vi "Tavle Save Conver to PD .vi"(8 "error in (no error)":errorcluster, 11 "SN":string="012345678911111111112") -> (0 "error out 2":errorcluster)   [LabVIEW 2019]
uses:
  Ctrl/Table Save.ctl
  Ctrl/MeasureDisplayTab.ctl
  Ctrl/PD Table Save Low Index.ctl
  Ctrl/PD Table Save Col Index.ctl
  <vilib>/Utility/sysdir.llb/System Directory Type.ctl
  <vilib>/Utility/file.llb/Read Delimited Spreadsheet (string).vi
  <vilib>/Utility/file.llb/Write Delimited Spreadsheet (string).vi
panel:
  out "硬體":string
  out "Read SN Table":string[][](array[string])
  out "first row":string[](array[string])
  out "all rows":string[][](array[string])
  out "error out":errorcluster
  in  "Read SN Table 2":string[][](array[string])
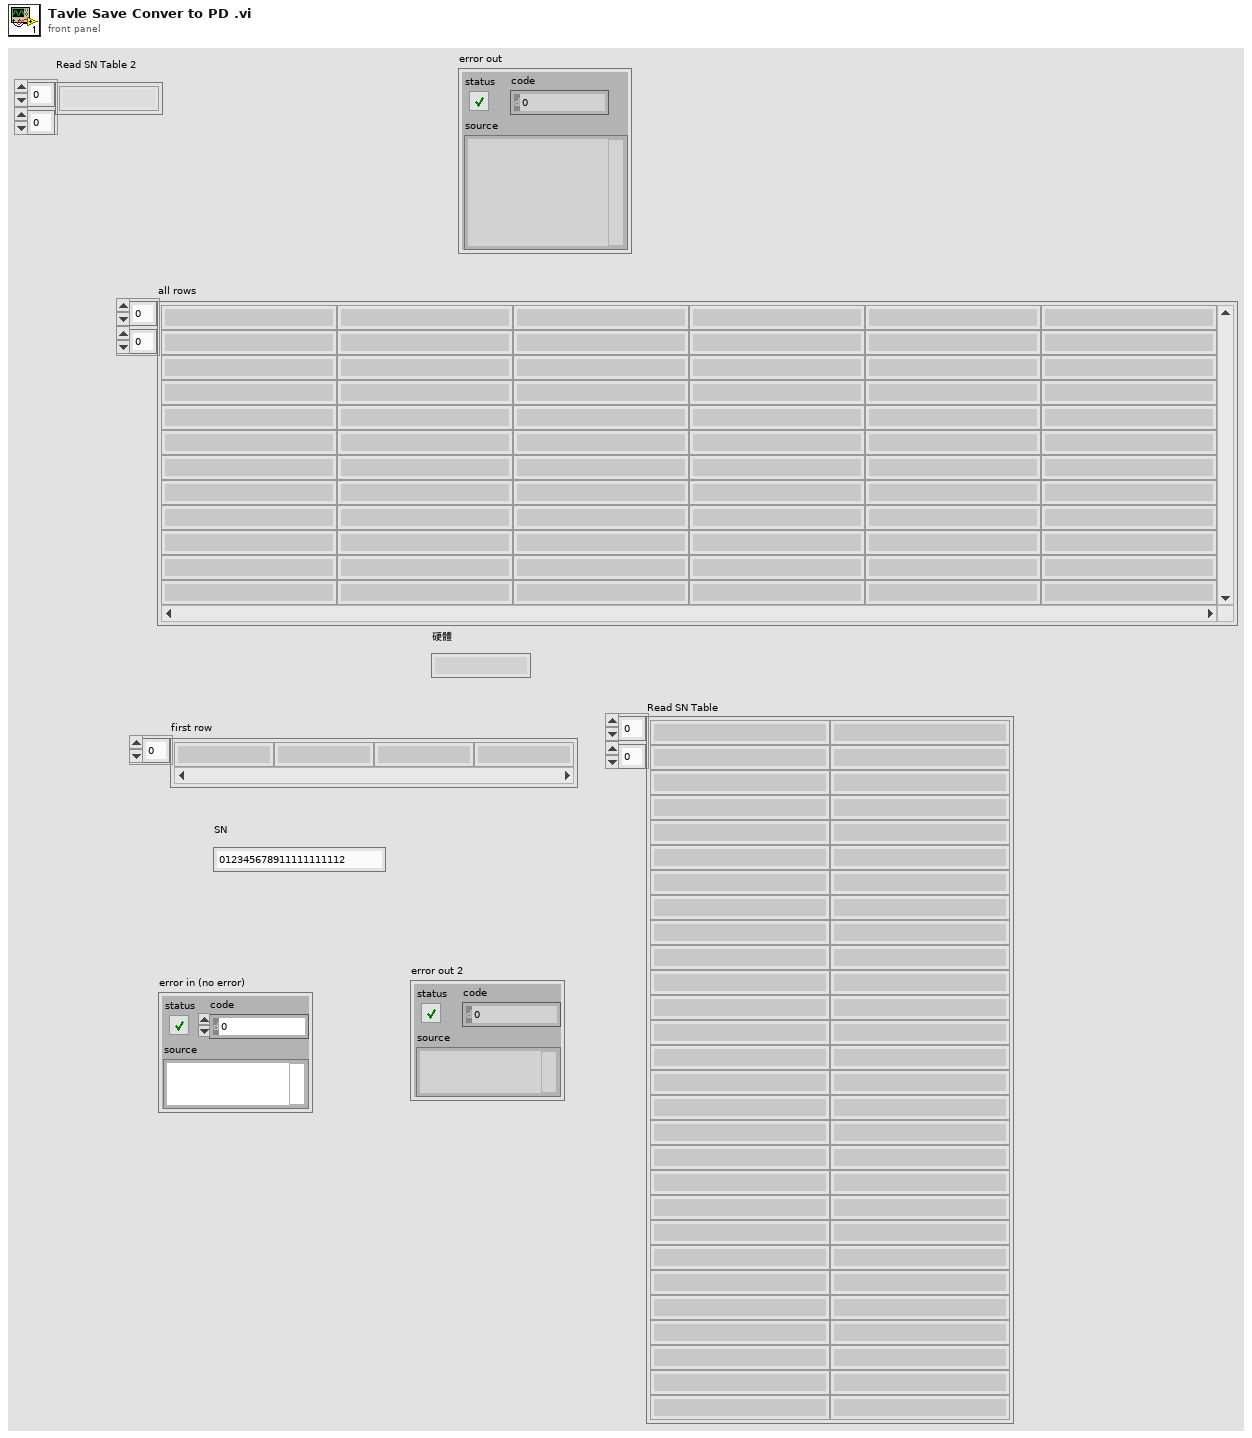
[diagram p1: front panel]
types:
  T1 = typedef "Table Save.ctl" = enum16{"initial", "Add", "Write", "Replace", "Delete", "REad", "RedTable", "Load"}
  T2 = typedef "MeasureDisplayTab.ctl" = enum16{"Tray Barcode", "PCBA BARCODE", "硬體(Tool初始化)", "company(Tool初始化)", "耗電流 uA(電流表)", "電池負載電壓", "晶片ID(Tool FORMAT)", "雷雕ID(TOOl scan、藍芽接收器)", "Format(Tool FORMAT)", "Programe(Tool Programe)", "MAC(藍芽接收器)", "ID(藍芽接收器)", "KPA(藍芽接收器)", "溫度(藍芽接收器)", "SENSOR電池電壓(藍芽接收器)", "RSSI(藍芽接收器)", "SensorType_315(FSK scan)", "FSKsnVol_315(FSK scan)", "FSKscanl_315(FSK scan)", "P_315(FSK scan)", "T_315(FSK scan)", "SensorType_433(ASK scan)", "ASKsnVol_433(ASK scan)", "ASKscan_433(ASK scan)", "P_433(ASK scan)", "T_433(ASK scan)", "測高Data"}
  T3 = typedef "PD Table Save Col Index.ctl" = enum16{"Col A", "Col B", "PCBA SN_C", "scan 半成品 ID_1_D", "半成品 Waste_Time_E", "半成品 Result_F", "半成品 DateTime_G", "433半成品 版本_H", "433半成品 company_I", "433半成品 FF_J", "433半成品 SensorType_K", "433半成品 BattVol_L", "433半成品 ASKsnVOL_M", "433半成品 ID_2_N", "433半成品 Format_O", "433半成品 Programe_P", "433半成品 ASKscan_Q", "433半成品 FSKscan_R", "433半成品 Batt_S", "433半成品 SN_T", "433半成品 Ptest_U", "433半成品 Ttest_V", "433半成品 P_W", "433半成品 T_X", "433半成品 結果_Y", "433半成品 箱號_Z", "不良代碼_AA", "電流_AB", "電池電壓_AC", "315半成品 版本_AD", "315半成品 company_AE", "315半成品 FF_AF", "315半成品 SensorType_AG", "315半成品 BattVol_AH", "315半成品 ASKsnVOL_AI", "315半成品 ID_2_AJ", "315半成品 Format_AK", "315半成品 Programe_AL", "315半成品 ASKscan_AM", "315半成品 FSKscan_AN", "315半成品 Batt_AO", "315半成品 SN_AP", "315半成品 Ptest_AQ", "315半成品 Ttest_AR", "315半成品 P_AS", "315半成品 T_AT"}
  T4 = typedef "PD Table Save Low Index.ctl" = enum16{"low 1", "low 2", "low 3", "low 4", "一般模式F", "一般模式P", "一般模式S", "low 8", "藍芽模式F", "藍芽模式P", "藍芽模式S"}
  T5 = typedef "System Directory Type.ctl" = i32
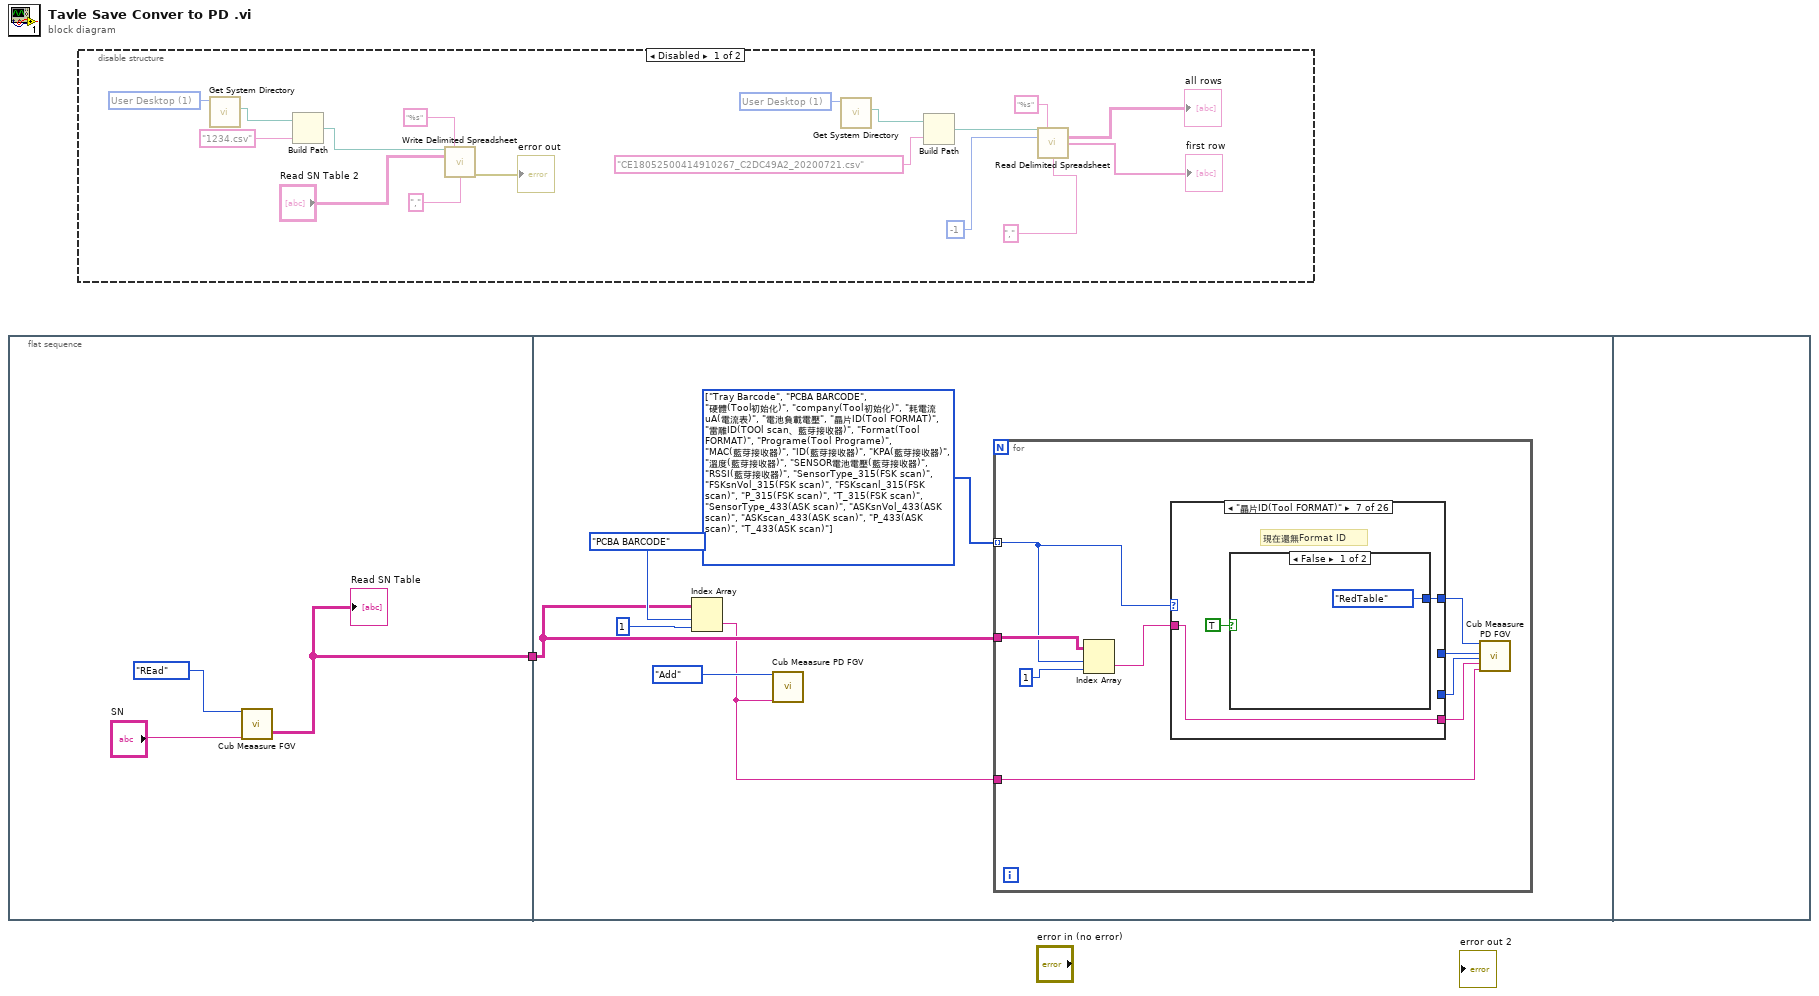
[diagram p0: block diagram]
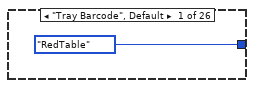
[diagram p3: hidden frame]
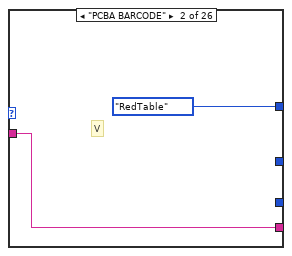
[diagram p4: hidden frame]
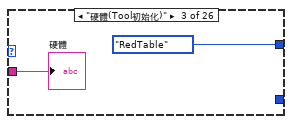
[diagram p5: hidden frame]
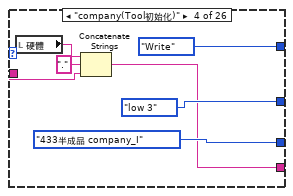
[diagram p6: hidden frame]
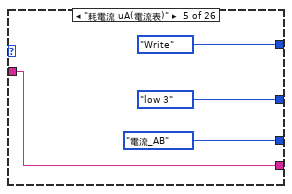
[diagram p7: hidden frame]
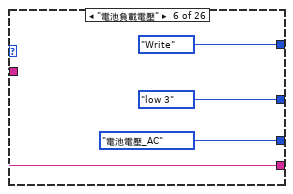
[diagram p8: hidden frame]
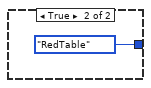
[diagram p9: hidden frame]
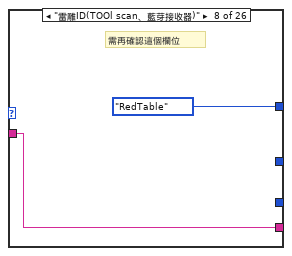
[diagram p10: hidden frame]
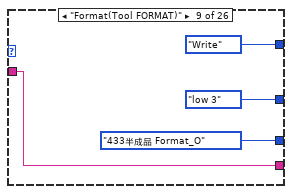
[diagram p11: hidden frame]
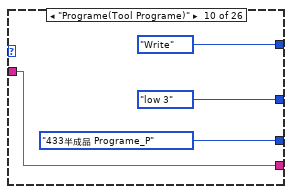
[diagram p12: hidden frame]
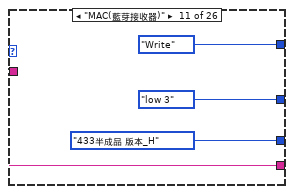
[diagram p13: hidden frame]
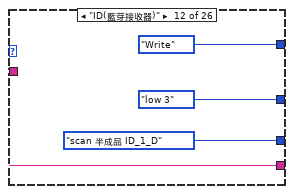
[diagram p14: hidden frame]
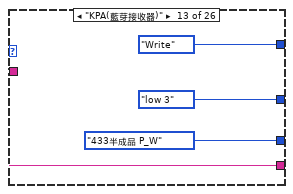
[diagram p15: hidden frame]
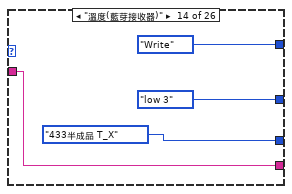
[diagram p16: hidden frame]
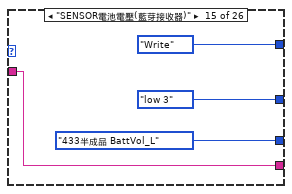
[diagram p17: hidden frame]
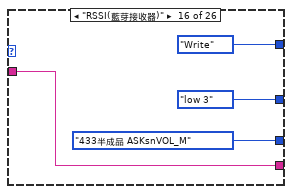
[diagram p18: hidden frame]
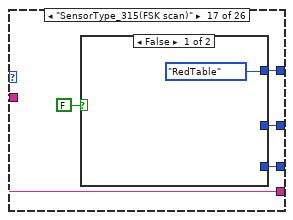
[diagram p19: hidden frame]
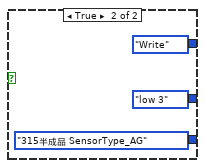
[diagram p20: hidden frame]
diagram:
  n1 = flat-sequence {
    tunnel: [w3] -> w1
    tunnel: w1 -> [w7]
    frame #0 {
      n2 = call "Cub Meaasure FGV.vi"("Action"=Table_Save."REad", "SN"="SN") -> ("Read SN Table"=w3:string[][])  [unwired: 10 in, 7 out]
      "Read SN Table" <- w3
    }
    frame #1 {
      w5 = T2[] [enum."Tray Barcode", enum."PCBA BARCODE", enum."硬體(Tool初始化)", enum."company(Tool初始化)", enum."耗電流 uA(電流表)", enum."電池負載電壓", enum."晶片ID(Tool FORMAT)", enum."雷雕ID(TOOl scan、藍芽接收器)", enum."Format(Tool FORMAT)", enum."Programe(Tool Programe)", enum."MAC(藍芽接收器)", enum."ID(藍芽接收器)", enum."KPA(藍芽接收器)", enum."溫度(藍芽接收器)", enum."SENSOR電池電壓(藍芽接收器)", enum."RSSI(藍芽接收器)", enum."SensorType_315(FSK scan)", enum."FSKsnVol_315(FSK scan)", enum."FSKscanl_315(FSK scan)", enum."P_315(FSK scan)", enum."T_315(FSK scan)", enum."SensorType_433(ASK scan)", enum."ASKsnVol_433(ASK scan)", enum."ASKscan_433(ASK scan)", enum."P_433(ASK scan)", enum."T_433(ASK scan)"] items=["Tray Barcode", "PCBA BARCODE", "硬體(Tool初始化)", "company(Tool初始化)", "耗電流 uA(電流表)", "電池負載電壓", "晶片ID(Tool FORMAT)", "雷雕ID(TOOl scan、藍芽接收器)", "Format(Tool FORMAT)", "Programe(Tool Programe)", "MAC(藍芽接收器)", "ID(藍芽接收器)", "KPA(藍芽接收器)", "溫度(藍芽接收器)", "SENSOR電池電壓(藍芽接收器)", "RSSI(藍芽接收器)", "SensorType_315(FSK scan)", "FSKsnVol_315(FSK scan)", "FSKscanl_315(FSK scan)", "P_315(FSK scan)", "T_315(FSK scan)", "SensorType_433(ASK scan)", "ASKsnVol_433(ASK scan)", "ASKscan_433(ASK scan)", "P_433(ASK scan)", "T_433(ASK scan)", "測高Data"]
      n3 = Index Array(array=w7, index (row)=MeasureDisplayTab."PCBA BARCODE" ("Save Index"), index (col)=1 ("disabled index (col)")) -> (element=w6:string)
      n4 = call "Cub Meaasure PD FGV.vi"("Action"=Table_Save."Add", "SN"=w6) -> ()  [unwired: 10 in, 8 out]
      n5 = for {
        tunnel: w7 -> [w17]
        tunnel: w5 -> [w14] mode=indexing
        tunnel: w6 -> [w11]
        n6 = Index Array(array=w17, index (row)=w14, index (col)=1 ("disabled index (col)")) -> (element=w15:string)
        n7 = case shown="\"晶片ID(Tool FORMAT)\"" w14 {
          tunnel: w15 -> [_ w22 w23 w26 w32 w36 w41 w45 w47 w51 w55 w59 w63 w67 w71 w75 w80 w89 w100 w111 w122 w133 w144 w154 w159 w170]
          tunnel: [_ _ _ PD_Table_Save_Low_Index."low 3" PD_Table_Save_Low_Index."low 3" PD_Table_Save_Low_Index."low 3" _ _ PD_Table_Save_Low_Index."low 3" PD_Table_Save_Low_Index."low 3" PD_Table_Save_Low_Index."low 3" PD_Table_Save_Low_Index."low 3" PD_Table_Save_Low_Index."low 3" PD_Table_Save_Low_Index."low 3" PD_Table_Save_Low_Index."low 3" PD_Table_Save_Low_Index."low 3" w82 w91 w102 w113 w124 w135 w146 PD_Table_Save_Low_Index."low 3" w161 w172] -> w19
          tunnel: [_ _ _ PD_Table_Save_Col_Index."433半成品 company_I" ("Save Col Index") PD_Table_Save_Col_Index."電流_AB" ("Save Col Index") PD_Table_Save_Col_Index."電池電壓_AC" ("Save Col Index") _ _ PD_Table_Save_Col_Index."433半成品 Format_O" ("Save Col Index") PD_Table_Save_Col_Index."433半成品 Programe_P" ("Save Col Index") PD_Table_Save_Col_Index."433半成品 版本_H" ("Save Col Index") PD_Table_Save_Col_Index."scan 半成品 ID_1_D" ("Save Col Index") PD_Table_Save_Col_Index."433半成品 P_W" ("Save Col Index") PD_Table_Save_Col_Index."433半成品 T_X" ("Save Col Index") PD_Table_Save_Col_Index."433半成品 BattVol_L" ("Save Col Index") PD_Table_Save_Col_Index."433半成品 ASKsnVOL_M" ("Save Col Index") w81 w90 w101 w112 w123 w134 w145 PD_Table_Save_Col_Index."433半成品 ASKscan_Q" ("Save Col Index") w160 w171] -> w18
          tunnel: [_ w22 _ w25 w32 w36 w41 w45 w47 w51 w55 w59 w63 w67 w71 w75 w80 w89 w100 w111 w122 w133 w144 w154 w159 w170] -> w12
          tunnel: [Table_Save."RedTable" ("Action") Table_Save."RedTable" ("Action") Table_Save."RedTable" ("Action") Table_Save."Write" ("Action") Table_Save."Write" ("Action") Table_Save."Write" ("Action") w42 Table_Save."RedTable" ("Action") Table_Save."Write" ("Action") Table_Save."Write" ("Action") Table_Save."Write" ("Action") Table_Save."Write" ("Action") Table_Save."Write" ("Action") Table_Save."Write" ("Action") Table_Save."Write" ("Action") Table_Save."Write" ("Action") w83 w92 w103 w114 w125 w136 w147 Table_Save."Write" ("Action") w162 w173] -> w13
          frame "Tray Barcode", Default {
          }
          frame "PCBA BARCODE" {
            # "V"
          }
          frame "硬體(Tool初始化)" {
            "硬體" <- w23
          }
          frame "company(Tool初始化)" {
            n8 = local read "硬體"() -> (w28:string)
            n9 = Concatenate Strings(w28, "." ("string"), w26) -> (w25:string)
          }
          frame "耗電流 uA(電流表)" {
          }
          frame "電池負載電壓" {
          }
          frame "晶片ID(Tool FORMAT)" {
            # "現在還無Format ID"
            n10 = case shown="False" TRUE {
              tunnel: [Table_Save."RedTable" ("Action") Table_Save."RedTable" ("Action")] -> w42
              frame False {
              }
              frame True {
              }
            }
          }
          frame "雷雕ID(TOOl scan、藍芽接收器)" {
            # "需再確認這個欄位"
          }
          frame "Format(Tool FORMAT)" {
          }
          frame "Programe(Tool Programe)" {
          }
          frame "MAC(藍芽接收器)" {
          }
          frame "ID(藍芽接收器)" {
          }
          frame "KPA(藍芽接收器)" {
          }
          frame "溫度(藍芽接收器)" {
          }
          frame "SENSOR電池電壓(藍芽接收器)" {
          }
          frame "RSSI(藍芽接收器)" {
          }
          frame "SensorType_315(FSK scan)" {
            n11 = case shown="False" FALSE {
              tunnel: [Table_Save."RedTable" ("Action") Table_Save."Write" ("Action")] -> w83
              tunnel: [_ PD_Table_Save_Low_Index."low 3"] -> w82
              tunnel: [_ PD_Table_Save_Col_Index."315半成品 SensorType_AG" ("Save Col Index")] -> w81
              frame False {
              }
              frame True {
              }
            }
          }
          frame "FSKsnVol_315(FSK scan)" {
            n12 = case shown="False" FALSE {
              tunnel: [Table_Save."RedTable" ("Action") Table_Save."Write" ("Action")] -> w92
              tunnel: [PD_Table_Save_Low_Index."low 3" PD_Table_Save_Low_Index."low 3"] -> w91
              tunnel: [PD_Table_Save_Col_Index."315半成品 ASKsnVOL_AI" ("Save Col Index") PD_Table_Save_Col_Index."315半成品 ASKsnVOL_AI" ("Save Col Index")] -> w90
              frame False {
              }
              frame True {
              }
            }
          }
          frame "FSKscanl_315(FSK scan)" {
            n13 = case shown="False" FALSE {
              tunnel: [Table_Save."RedTable" ("Action") Table_Save."Write" ("Action")] -> w103
              tunnel: [PD_Table_Save_Low_Index."low 3" PD_Table_Save_Low_Index."low 3"] -> w102
              tunnel: [PD_Table_Save_Col_Index."315半成品 FSKscan_AN" ("Save Col Index") PD_Table_Save_Col_Index."315半成品 FSKscan_AN" ("Save Col Index")] -> w101
              frame False {
              }
              frame True {
              }
            }
          }
          frame "P_315(FSK scan)" {
            n14 = case shown="False" FALSE {
              tunnel: [Table_Save."RedTable" ("Action") Table_Save."Write" ("Action")] -> w114
              tunnel: [PD_Table_Save_Low_Index."low 3" PD_Table_Save_Low_Index."low 3"] -> w113
              tunnel: [PD_Table_Save_Col_Index."315半成品 P_AS" ("Save Col Index") PD_Table_Save_Col_Index."315半成品 P_AS" ("Save Col Index")] -> w112
              frame False {
              }
              frame True {
              }
            }
          }
          frame "T_315(FSK scan)" {
            n15 = case shown="False" FALSE {
              tunnel: [Table_Save."RedTable" ("Action") Table_Save."Write" ("Action")] -> w125
              tunnel: [PD_Table_Save_Low_Index."low 3" PD_Table_Save_Low_Index."low 3"] -> w124
              tunnel: [PD_Table_Save_Col_Index."315半成品 T_AT" ("Save Col Index") PD_Table_Save_Col_Index."315半成品 T_AT" ("Save Col Index")] -> w123
              frame False {
              }
              frame True {
              }
            }
          }
          frame "SensorType_433(ASK scan)" {
            n16 = case shown="False" TRUE {
              tunnel: [Table_Save."RedTable" ("Action") Table_Save."Write" ("Action")] -> w136
              tunnel: [PD_Table_Save_Low_Index."low 3" PD_Table_Save_Low_Index."low 3"] -> w135
              tunnel: [PD_Table_Save_Col_Index."433半成品 SensorType_K" ("Save Col Index") PD_Table_Save_Col_Index."433半成品 SensorType_K" ("Save Col Index")] -> w134
              frame False {
              }
              frame True {
              }
            }
          }
          frame "ASKsnVol_433(ASK scan)" {
            n17 = case shown="False" FALSE {
              tunnel: [Table_Save."RedTable" ("Action") Table_Save."Write" ("Action")] -> w147
              tunnel: [PD_Table_Save_Low_Index."low 3" PD_Table_Save_Low_Index."low 3"] -> w146
              tunnel: [PD_Table_Save_Col_Index."433半成品 ASKsnVOL_M" ("Save Col Index") PD_Table_Save_Col_Index."433半成品 ASKsnVOL_M" ("Save Col Index")] -> w145
              frame False {
              }
              frame True {
              }
            }
          }
          frame "ASKscan_433(ASK scan)" {
          }
          frame "P_433(ASK scan)" {
            # "藍芽模式時不存"
            n18 = case shown="False" FALSE {
              tunnel: [Table_Save."RedTable" ("Action") Table_Save."Write" ("Action")] -> w162
              tunnel: [PD_Table_Save_Low_Index."low 3" PD_Table_Save_Low_Index."low 3"] -> w161
              tunnel: [PD_Table_Save_Col_Index."433半成品 P_W" ("Save Col Index") PD_Table_Save_Col_Index."433半成品 P_W" ("Save Col Index")] -> w160
              frame False {
              }
              frame True {
              }
            }
          }
          frame "T_433(ASK scan)" {
            # "藍芽模式時不存"
            n19 = case shown="False" FALSE {
              tunnel: [Table_Save."RedTable" ("Action") Table_Save."Write" ("Action")] -> w173
              tunnel: [PD_Table_Save_Low_Index."low 3" PD_Table_Save_Low_Index."low 3"] -> w172
              tunnel: [PD_Table_Save_Col_Index."433半成品 T_X" ("Save Col Index") PD_Table_Save_Col_Index."433半成品 T_X" ("Save Col Index")] -> w171
              frame False {
              }
              frame True {
              }
            }
          }
        }
        n20 = call "Cub Meaasure PD FGV.vi"("Action"=w13, "Save low Index"=w19, "Save Col Index"=w18, "DataIn"=w12, "SN"=w11) -> ()  [unwired: 7 in, 8 out]
      }
    }
    frame #2 {
    }
  }
  n21 = disable-structure shown="Disabled" {
    frame Disabled {
      w183 = T5 1 items=["User Home"=0, "User Desktop"=1, "User Documents"=2, "User Application Data"=3, "User Preferences"=4, "User Temporary"=5, "Public Documents"=6, "Public Application Data"=7, "Public Preferences"=8, "Public Cache"=13, "System Core Libraries"=9, "System Installed Libraries"=10, "Application Files"=11, "Boot Volume Root"=12] ("system directory type")
      w192 = T5 1 items=["User Home"=0, "User Desktop"=1, "User Documents"=2, "User Application Data"=3, "User Preferences"=4, "User Temporary"=5, "Public Documents"=6, "Public Application Data"=7, "Public Preferences"=8, "Public Cache"=13, "System Core Libraries"=9, "System Installed Libraries"=10, "Application Files"=11, "Boot Volume Root"=12] ("system directory type")
      n22 = call <vilib>:"Get System Directory.vi"("system directory type"=w192) -> ("system directory"=w195:path)  [unwired: 10 in]
      n23 = Build Path(base path=w195, name or relative path="1234.csv") -> (appended path=w196:path)
      n24 = call-poly <vilib>:"Write Delimited Spreadsheet.vi"("file path (dialog if empty)"=w196, "format (%s)"="%s", "2D data"="Read SN Table 2", "delimiter (\\t)"="," ("delimiter (\\t)")) -> ("error out"=→"error out":errorcluster)  [unwired: 10 in, 1 out]
      n25 = call <vilib>:"Get System Directory.vi"("system directory type"=w183) -> ("system directory"=w182:path)  [unwired: 10 in]
      n26 = Build Path(base path=w182, name or relative path="CE18052500414910267_C2DC49A2_20200721.csv") -> (appended path=w181:path)
      n27 = call-poly <vilib>:"Read Delimited Spreadsheet.vi"("file path (dialog if empty)"=w181, "format (%s)"="%s", "number of rows (all:-1)"=-1, "delimiter (\\t)"="," ("delimiter (\\t)")) -> ("all rows"=→"all rows":string[][], "first row"=→"first row":string[])  [unwired: 6 in, 4 out]
    }
    frame Enabled {
    }
  }
